vi "cameraParameters.vi"(2 "Camera Device  IN":T2, 3 "Camera Parameters":refnum<vi>, 4 "Selector":refnum<vi>, 5 "Stream?":refnum<vi>) -> (0 "Camera Device OUT":T1, 1 "Stream? OUT":bool)   [LabVIEW 2010]
uses:
  <vilib>/addons/PixeLINK/Low Level Functions/CAMERA_FEATURES.llb/TDPU-CameraFeatures-PixelFormat.ctl
  <vilib>/Utility/error.llb/DialogType.ctl
  <vilib>/addons/PixeLINK/Low Level Functions/CAMERA_FEATURES.llb/TDPU-CameraFeatures-FeatureFlags.ctl
  <vilib>/addons/PixeLINK/Low Level Functions/CAMERA_FEATURES.llb/TDPU-CameraFeatures-FeatureIds.ctl
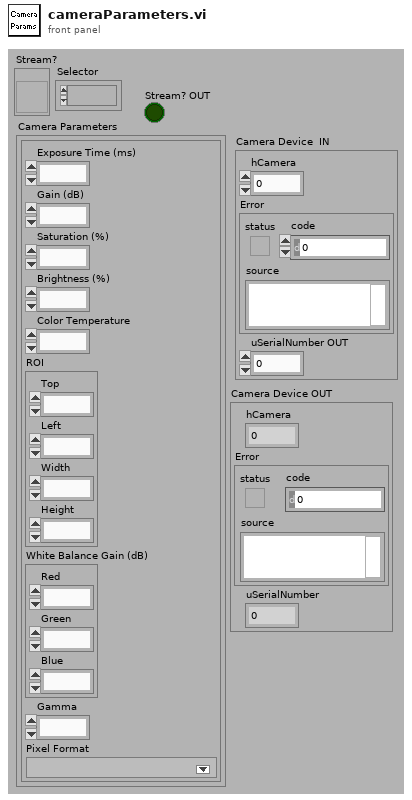
[diagram p1: front panel]
types:
  T1 = cluster{"hCamera":u32, "Error":errorcluster, "uSerialNumber":u32}
  T2 = cluster{"hCamera":u32, "Error":errorcluster, "uSerialNumber OUT":u32}
  T3 = typedef "TDPU-CameraFeatures-PixelFormat.ctl" = u16
  T4 = cluster{"Selector":u16, "Stream?":bool, "Camera Parameters":cluster{"Exposure Time (ms)":u32, "Gain (dB)":dbl, "Saturation (%)":dbl, "Brightness (%)":dbl, "Color Temperature":dbl, "ROI":cluster{"Top":i32, "Left":i32, "Width":i32, "Height":i32}, "White Balance Gain (dB)":cluster{"Red":dbl, "Green":dbl, "Blue":dbl}, "Gamma":dbl, "Pixel Format":T3}}
  T5 = cluster{"Exposure Time (ms)":u32, "Gain (dB)":dbl, "Saturation (%)":dbl, "Brightness (%)":dbl, "Color Temperature":dbl, "ROI":cluster{"Top":i32, "Left":i32, "Width":i32, "Height":i32}, "White Balance Gain (dB)":cluster{"Red":dbl, "Green":dbl, "Blue":dbl}, "Gamma":dbl, "Pixel Format":T3}
  T6 = cluster{"Exposure Time (ms)":dbl, "Gain (dB)":dbl, "Saturation (%)":dbl, "Brightness (%)":dbl, "Color Temperature":dbl, "ROI":cluster{"Top":i32, "Left":i32, "Width":i32, "Height":i32}, "White Balance Gain (dB)":cluster{"Red":dbl, "Green":dbl, "Blue":dbl}, "Gamma":dbl, "Pixel Format":T3}
  T7 = typedef "DialogType.ctl" = u16
  T8 = enum16{"Exposure Time (ms)", "Gain (dB)", "Saturation (%)", "Brightness (%)", "Color Temperature (%)", "ROI", "White Balance Gain (dB)", "Gamma", "Pixel Format", "Selector", "Stream", "Nothing"}[]
  T9 = typedef "TDPU-CameraFeatures-FeatureFlags.ctl" = u32
  T10 = typedef "TDPU-CameraFeatures-FeatureIds.ctl" = u32
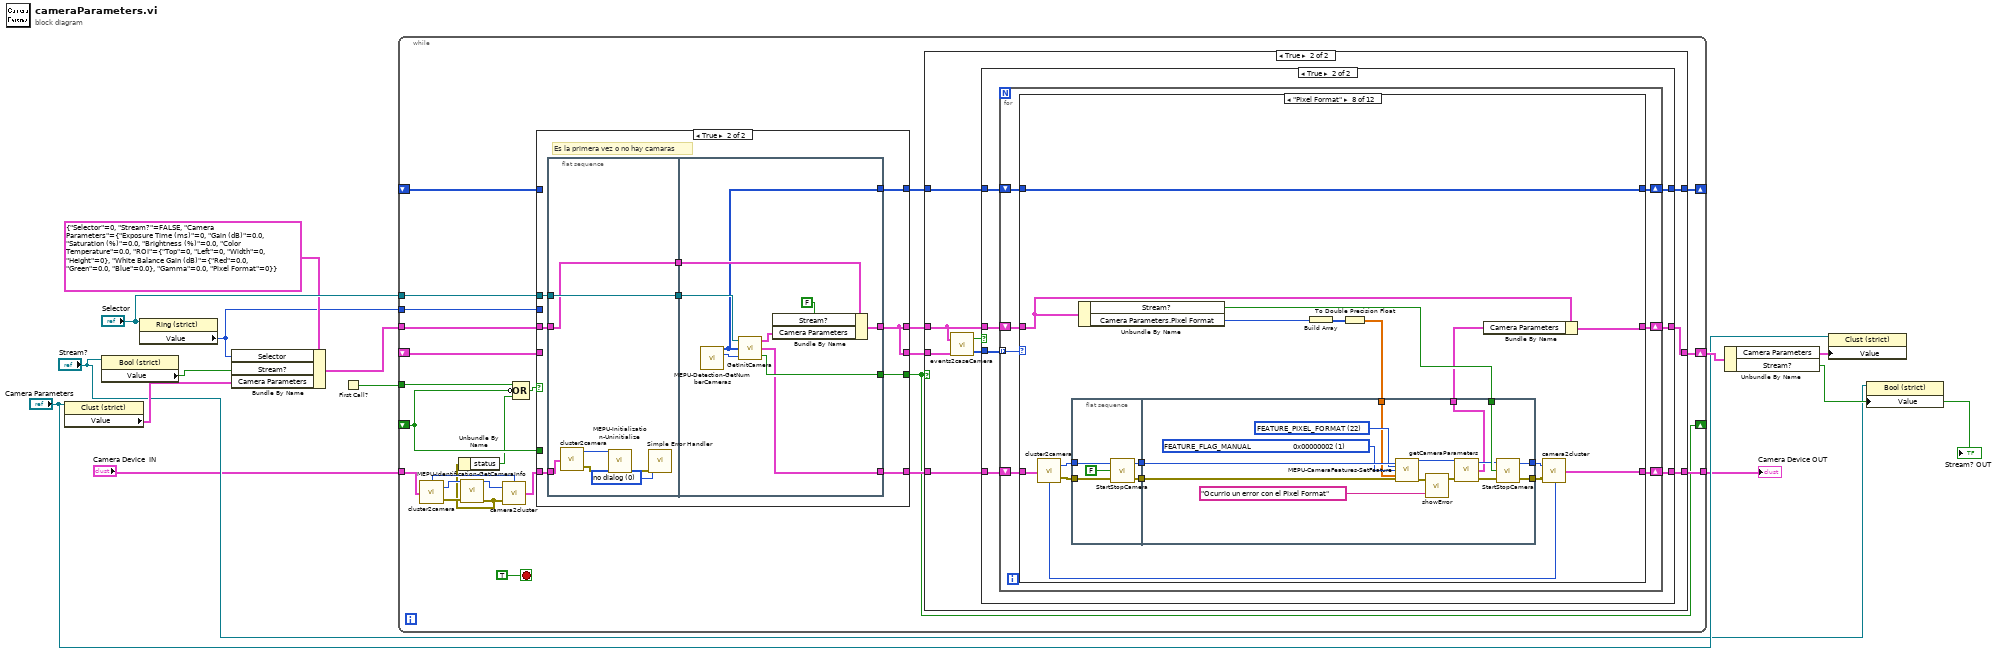
[diagram p0: block diagram]
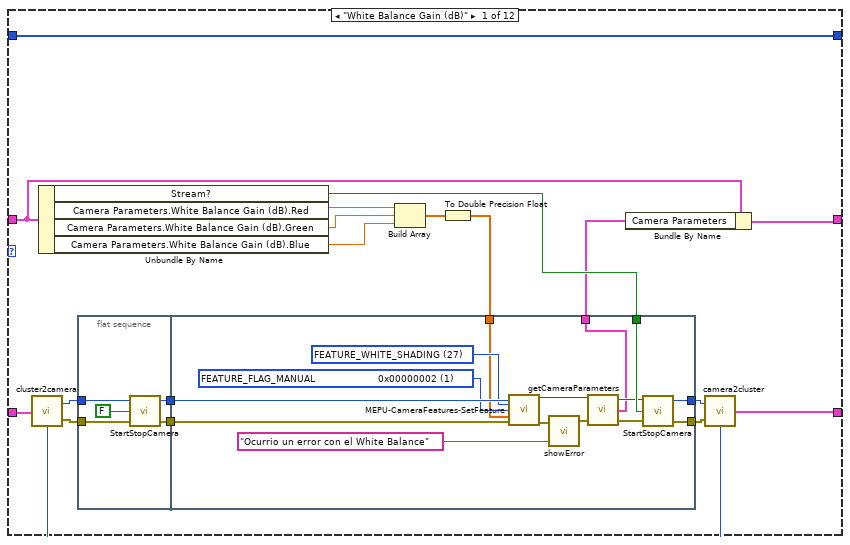
[diagram p4: hidden frame]
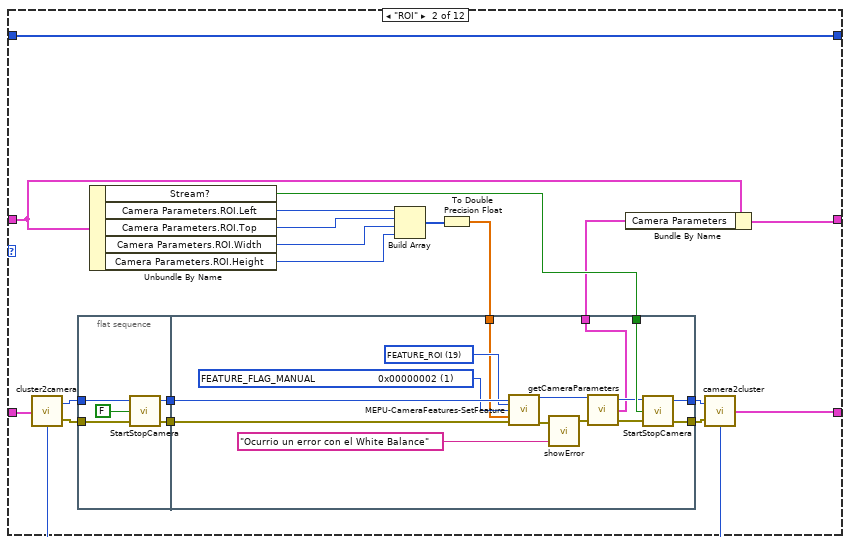
[diagram p5: hidden frame]
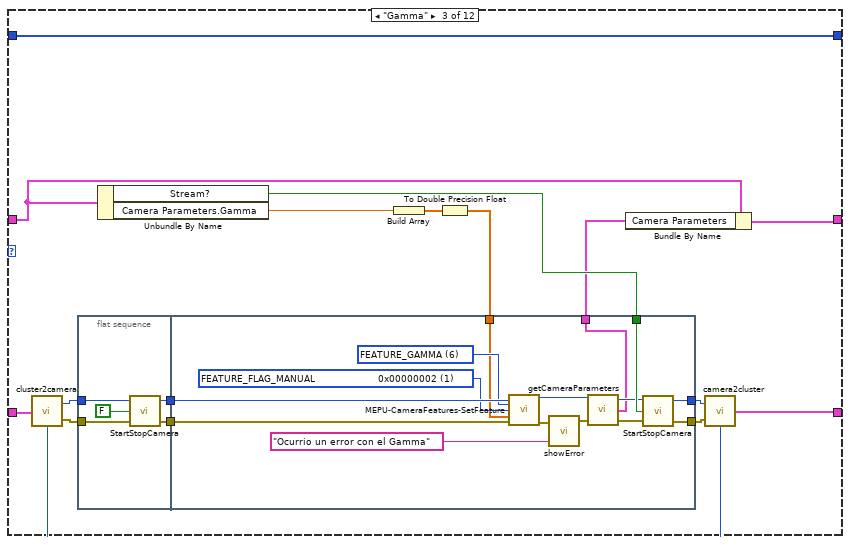
[diagram p6: hidden frame]
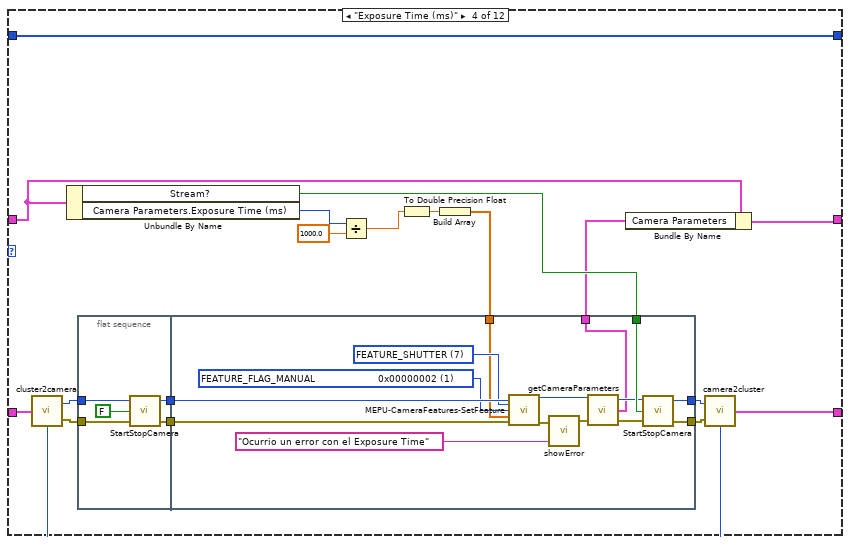
[diagram p7: hidden frame]
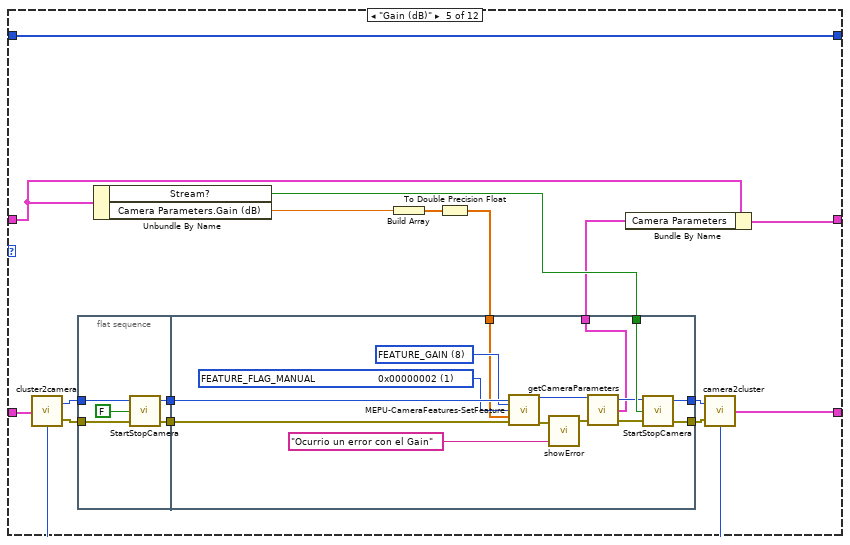
[diagram p8: hidden frame]
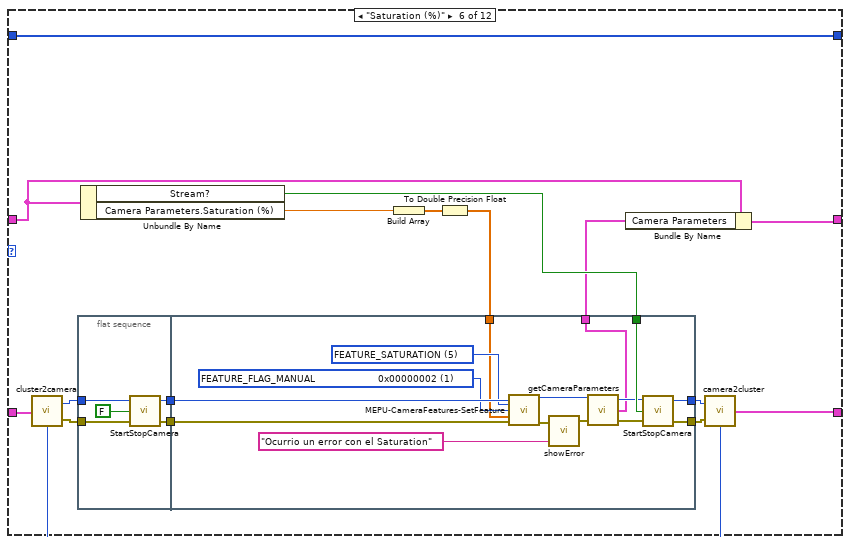
[diagram p9: hidden frame]
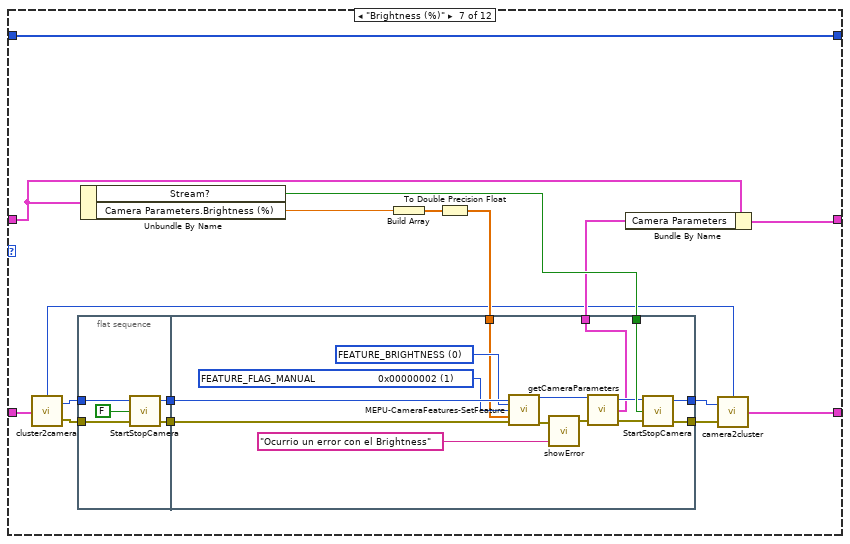
[diagram p10: hidden frame]
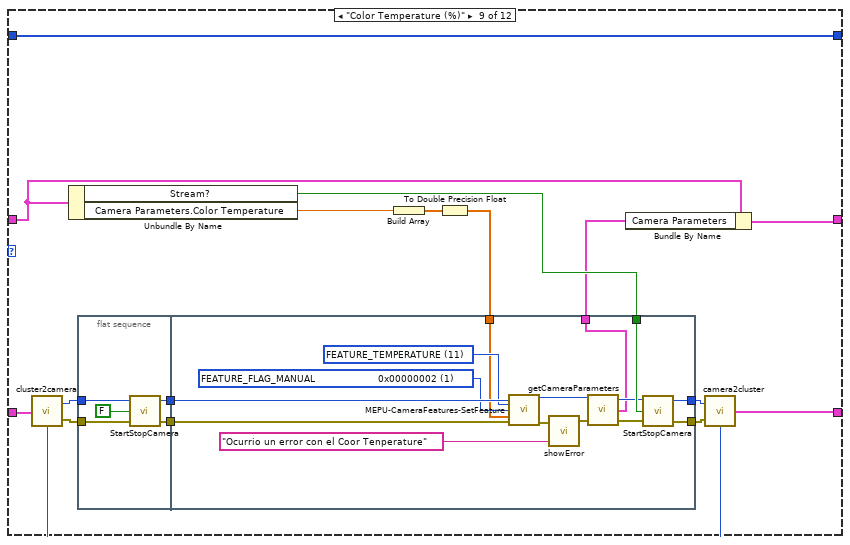
[diagram p11: hidden frame]
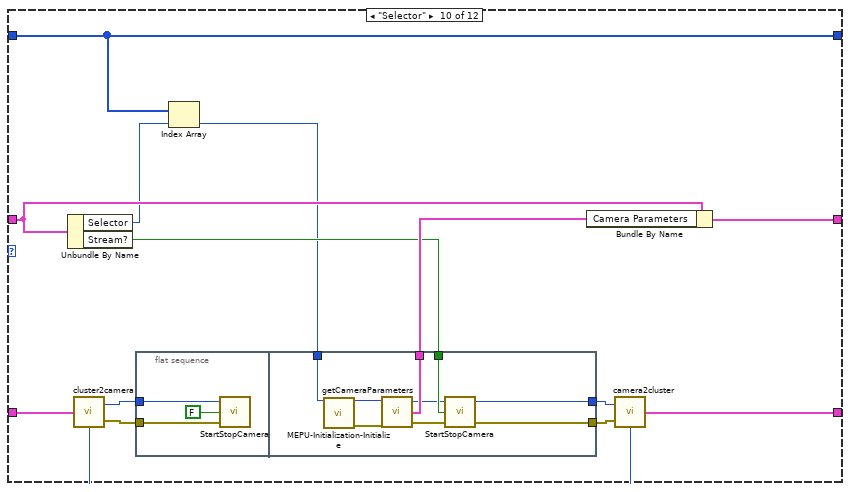
[diagram p12: hidden frame]
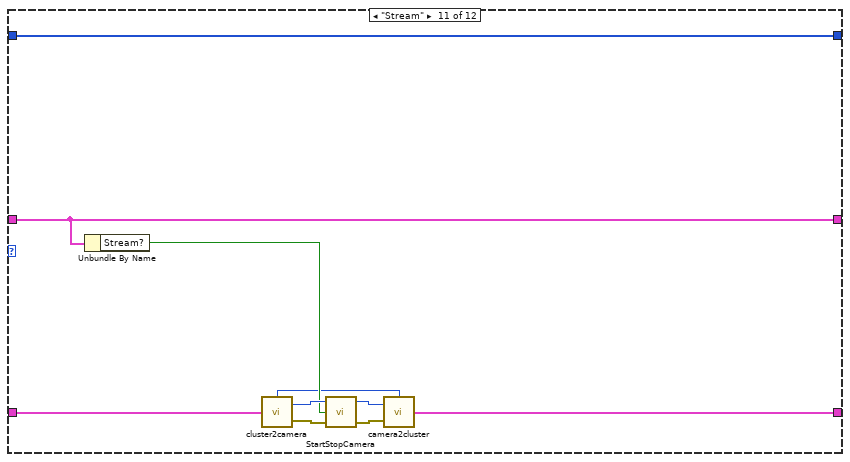
[diagram p13: hidden frame]
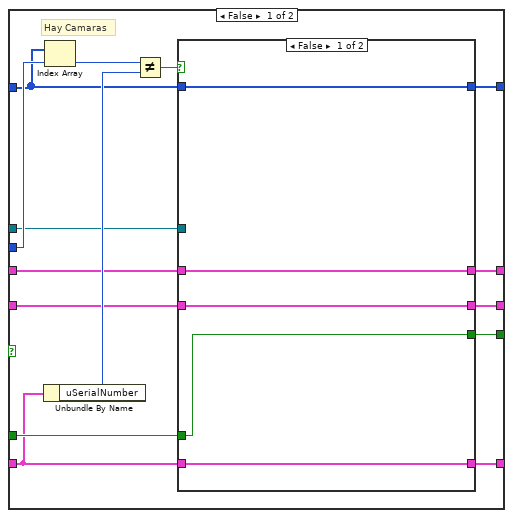
[diagram p15: hidden frame]
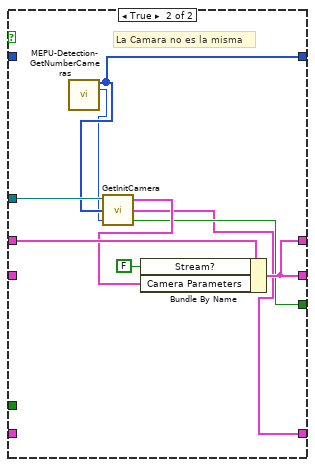
[diagram p16: hidden frame]
diagram:
  n1 = property class="Clust (strict)"(reference="Camera Parameters") -> ("Value"=w7:T5)  [unwired: 1 in, 2 out]
  n2 = property class="Bool (strict)"(reference="Stream?") -> ("Value"=w6:bool)  [unwired: 1 in, 2 out]
  n3 = property class="Ring (strict)"(reference="Selector") -> ("Value"=w3:u16)  [unwired: 1 in, 2 out]
  n4 = Bundle By Name(cluster=T4 {"Selector"=0, "Stream?"=FALSE, "Camera Parameters"={"Exposure Time (ms)"=0, "Gain (dB)"=0.0, "Saturation (%)"=0.0, "Brightness (%)"=0.0, "Color Temperature"=0.0, "ROI"={"Top"=0, "Left"=0, "Width"=0, "Height"=0}, "White Balance Gain (dB)"={"Red"=0.0, "Green"=0.0, "Blue"=0.0}, "Gamma"=0.0, "Pixel Format"=0}}, "Selector"=w3, "Stream?"=w6, "Camera Parameters"=w7) -> (w13:T4)
  n5 = First Call?() -> (First Call?: T/F=w14:bool)
  n6 = while {
    tunnel: w13 -> [w35]
    shift-right: [w38] -> w12
    shift-left: _ -> [w34]
    tunnel: "Camera Device  IN" -> [w18]
    tunnel: [w37] -> w1
    tunnel: w14 -> [w25]
    tunnel: "Selector" -> [w31]
    shift-right: [w27] -> _
    shift-left: _ -> [w30]
    shift-right: [w26] -> _
    shift-left: _ -> [w23]
    tunnel: w3 -> [w24]
    stop <- TRUE stop-if-true
    n7 = call "cluster2camera.vi"("Camera Device IN"=w18) -> ("Error OUT"=w22:errorcluster, "hCamera OUT"=w21:u32, "uSerialNumber OUT"=w19:u32)  [unwired: 2 in]
    n8 = call <vilib>:"MEPU-Identification-GetCameraInfo.vi"("hCamera IN"=w21, "Error IN"=w22) -> ("hCamera OUT"=w20:u32, "Error OUT"=w16:errorcluster)  [unwired: 11 in, 1 out]
    n9 = Unbundle By Name(w16) -> ("status"=w15:bool)
    n10 = call "camera2cluster.vi"("uSerialNumber IN"=w19, "Error IN"=w16, "hCamera IN"=w20) -> ("Camera Device OUT"=w17:T1)
    n11 = Compound Arithmetic op=OR(w25, invert w23, w15) -> (w29:bool)
    n12 = case shown="True" w29 {
      tunnel: [w458 w477] -> w28
      tunnel: [w456 w478] -> w36
      tunnel: w35 -> [w455 w480]
      tunnel: w34 -> [w453 _]
      tunnel: [w454 w478] -> w33
      tunnel: [w450 w481] -> w32
      tunnel: w17 -> [w449 w485]
      tunnel: w30 -> [w457 _]
      tunnel: [w452 w482] -> w26
      tunnel: w31 -> [w448 w483]
      tunnel: w24 -> [w462 _]
      tunnel: w23 -> [w451 _]
      frame False {
        # "Hay Camaras"
        n13 = Unbundle By Name(w449) -> ("uSerialNumber"=w460:u32)
        n14 = Index Array(array=w457, index=w462) -> (element=w461:u32)
        n15 = Not Equal?(x=w461, y=w460) -> (x != y?=w459:bool)
        n16 = case shown="False" w459 {
          tunnel: [w463 w475] -> w458
          tunnel: w457 -> [w463 _]
          tunnel: [w464 w472] -> w456
          tunnel: w455 -> [w464 w473]
          tunnel: [w465 w472] -> w454
          tunnel: w453 -> [w465 _]
          tunnel: [w466 w469] -> w452
          tunnel: w451 -> [w466 _]
          tunnel: [w467 w468] -> w450
          tunnel: w449 -> [w467 _]
          tunnel: w448 -> [_ w476]
          frame False {
          }
          frame True {
            # "La Camara no es la misma"
            n17 = call <vilib>:"MEPU-Detection-GetNumberCameras.vi"() -> ("LV_SerialNumbers OUT"=w475:u32[], "LV_NumberSerial OUT"=w474:u32)  [unwired: 13 in, 1 out]
            n18 = call "GetInitCamera.vi"("LV_NumberSerial IN"=w474, "LV_SerialNumbers IN"=w475, "Selector"=w476) -> ("Hay Camaras?"=w469:bool, "Camera Device OUT"=w468:T2, "Camera Parameters OUT"=w470:T6)
            n19 = Bundle By Name(cluster=w473, "Stream?"=FALSE, "Camera Parameters"=w470) -> (w472:T4)
          }
        }
      }
      frame True {
        # "Es la primera vez o no hay camaras"
        n20 = flat-sequence {
          tunnel: w485 -> [w488]
          tunnel: [w487] -> w484
          tunnel: w483 -> [w487]
          tunnel: w480 -> [w486]
          tunnel: [w486] -> w479
          tunnel: w484 -> [w500]
          tunnel: [w498] -> w482
          tunnel: [w497] -> w481
          tunnel: w479 -> [w495]
          tunnel: [w494] -> w478
          tunnel: [w493] -> w477
          frame #0 {
            w489 = T7 0 items=["no dialog", "OK message", "continue or stop message", "OK message + warnings", "continue/stop + warnings"] ("type of dialog (OK msg:1)")
            n21 = call "cluster2camera.vi"("Camera Device IN"=w488) -> ("Error OUT"=w492:errorcluster, "hCamera OUT"=w491:u32)  [unwired: 2 in, 1 out]
            n22 = call <vilib>:"MEPU-Initialization-Uninitialize.vi"("hCamera IN"=w491, "Error IN"=w492) -> ("Error OUT"=w490:errorcluster)  [unwired: 13 in]
            n23 = call <vilib>:"Simple Error Handler.vi"("type of dialog (OK msg:1)"=w489, "error in (no error)"=w490) -> ()  [unwired: 3 in, 5 out]
          }
          frame #1 {
            n24 = call <vilib>:"MEPU-Detection-GetNumberCameras.vi"() -> ("LV_SerialNumbers OUT"=w493:u32[], "LV_NumberSerial OUT"=w499:u32)  [unwired: 13 in, 1 out]
            n25 = call "GetInitCamera.vi"("LV_NumberSerial IN"=w499, "LV_SerialNumbers IN"=w493, "Selector"=w500) -> ("Hay Camaras?"=w498:bool, "Camera Device OUT"=w497:T2, "Camera Parameters OUT"=w496:T6)
            n26 = Bundle By Name(cluster=w495, "Stream?"=FALSE, "Camera Parameters"=w496) -> (w494:T4)
          }
        }
      }
    }
    n27 = case shown="True" w26 {
      tunnel: [w42 w50] -> w38
      tunnel: [w41 w48] -> w37
      tunnel: w28 -> [w40 w47]
      tunnel: w36 -> [w42 w46]
      tunnel: w33 -> [_ w45]
      tunnel: w32 -> [w41 w44]
      tunnel: [w40 w43] -> w27
      frame False {
      }
      frame True {
        n28 = call "events2caseCamera.vi"("Camara Controls Old"=w45, "Camara Controls New"=w46) -> ("Cameara Cambio Array"=w49:T8, "Camara Cambio?"=w51:bool)
        n29 = case shown="True" w51 {
          tunnel: [w54 w59] -> w50
          tunnel: w46 -> [w54 w60]
          tunnel: w49 -> [_ w61]
          tunnel: w44 -> [w53 w58]
          tunnel: [w53 w57] -> w48
          tunnel: w47 -> [w52 w56]
          tunnel: [w52 w55] -> w43
          frame False {
          }
          frame True {
            n30 = for {
              tunnel: w61 -> [w68] mode=indexing
              shift-right: [w66] -> w59
              shift-left: w60 -> [w67]
              shift-right: [w64] -> w57
              shift-left: w58 -> [w65]
              shift-right: [w63] -> w55
              shift-left: w56 -> [w62]
              n31 = case shown="\"Pixel Format\"" w68 {
                tunnel: w67 -> [w79 w119 w156 w195 w232 w269 w308 w343 w380 w421 w443 w447]
                tunnel: [w80 w120 w157 w196 w233 w270 w309 w344 w381 w422 w443 w447] -> w66
                tunnel: w65 -> [w71 w108 w150 w186 w225 w262 w299 w336 w374 w411 w437 w446]
                tunnel: [w70 w109 w149 w187 w226 w263 w300 w337 w372 w410 w436 w446] -> w64
                tunnel: [w74 w114 w153 w193 w229 w266 w305 w340 w377 w415 w444 w445] -> w63
                tunnel: w62 -> [w74 w114 w153 w193 w229 w266 w305 w340 w377 w415 w444 w445]
                frame "White Balance Gain (dB)" {
                  n32 = call "cluster2camera.vi"("Camera Device IN"=w71) -> ("Error OUT"=w84:errorcluster, "hCamera OUT"=w85:u32, "uSerialNumber OUT"=w69:u32)  [unwired: 2 in]
                  n33 = Unbundle By Name(w79) -> ("Stream?"=w81:bool, "Camera Parameters.White Balance Gain (dB).Red"=w78:dbl, "Camera Parameters.White Balance Gain (dB).Green"=w77:dbl, "Camera Parameters.White Balance Gain (dB).Blue"=w76:dbl)
                  n34 = flat-sequence {
                    tunnel: w85 -> [w91]
                    tunnel: w84 -> [w90]
                    tunnel: [w89] -> w87
                    tunnel: [w88] -> w86
                    tunnel: w81 -> [w107]
                    tunnel: [w106] -> w83
                    tunnel: [w105] -> w82
                    tunnel: w87 -> [w104]
                    tunnel: w86 -> [w103]
                    tunnel: [w97] -> w75
                    tunnel: w72 -> [w96]
                    frame #0 {
                      n35 = call "StartStopCamera.vi"("Error IN"=w90, "Camara ON?"=FALSE, "hCamera IN"=w91) -> ("Error OUT"=w88:errorcluster, "hCamera OUT"=w89:u32)  [unwired: 1 in]
                    }
                    frame #1 {
                      w101 = T9 1 items=["FEATURE_FLAG_PRESENCE                 0x00000001", "FEATURE_FLAG_MANUAL                     0x00000002", "FEATURE_FLAG_AUTO                         0x00000004", "FEATURE_FLAG_ONEPUSH                   0x00000008", "FEATURE_FLAG_OFF                            0x00000010", "FEATURE_FLAG_DESC_SUPPORTED    0x00000020", "FEATURE_FLAG_READ_ONLY               0x00000040"] ("uFlags IN")
                      w102 = T10 27 items=["FEATURE_BRIGHTNESS", "FEATURE_EXPOSURE", "FEATURE_SHARPNESS", "FEATURE_WHITE_BAL", "FEATURE_HUE", "FEATURE_SATURATION", "FEATURE_GAMMA", "FEATURE_SHUTTER", "FEATURE_GAIN", "FEATURE_IRIS", "FEATURE_FOCUS", "FEATURE_TEMPERATURE", "FEATURE_TRIGGER", "FEATURE_ZOOM", "FEATURE_PAN", "FEATURE_TILT", "FEATURE_OPT_FILTER", "FEATURE_GPIO", "FEATURE_FRAME_RATE", "FEATURE_ROI", "FEATURE_FLIP", "FEATURE_PIXEL_ADDRESSING", "FEATURE_PIXEL_FORMAT", "FEATURE_EXTENDED_SHUTTER", "FEATURE_AUTO_ROI", "FEATURE_LOOKUP_TABLE", "FEATURE_MEMORY_CHANNEL", "FEATURE_WHITE_SHADING", "FEATURE_ROTATE", "FEATURE_IMAGER_CLK_DIVISOR", "FEATURE_TRIG_WITH_CNTRLD_LIGHT", "FEATURE_MAX_PIXEL_SIZE"] ("uFeatureId IN")
                      n36 = call <vilib>:"MEPU-CameraFeatures-SetFeature.vi"("hCamera IN"=w104, "uFeatureId IN"=w102, "uFlags IN"=w101, "pParms IN"=w96, "Error IN"=w103) -> ("hCamera OUT"=w100:u32, "Error OUT"=w95:errorcluster)  [unwired: 8 in, 1 out]
                      n37 = call "showError.vi"("message"="Ocurrio un error con el White Balance", "Error IN"=w95) -> ("Error OUT"=w94:errorcluster)  [unwired: 3 in]
                      n38 = call "getCameraParameters.vi"("Error IN"=w94, "hCamera IN"=w100) -> ("Error OUT"=w98:errorcluster, "Camera Parameters"=w97:T6, "hCamera OUT"=w99:u32)  [unwired: 1 in]
                      n39 = call "StartStopCamera.vi"("Error IN"=w98, "Camara ON?"=w107, "hCamera IN"=w99) -> ("Error OUT"=w105:errorcluster, "hCamera OUT"=w106:u32)  [unwired: 1 in]
                    }
                  }
                  n40 = Build Array(w78, w77, w76) -> (w73:dbl[])
                  n41 = To Double Precision Float(number=w73) -> (double precision float=w72:dbl[])
                  n42 = Bundle By Name(cluster=w79, "Camera Parameters"=w75) -> (w80:T4)
                  n43 = call "camera2cluster.vi"("uSerialNumber IN"=w69, "Error IN"=w82, "hCamera IN"=w83) -> ("Camera Device OUT"=w70:T1)
                }
                frame "ROI" {
                  n44 = call "cluster2camera.vi"("Camera Device IN"=w108) -> ("Error OUT"=w124:errorcluster, "hCamera OUT"=w125:u32, "uSerialNumber OUT"=w110:u32)  [unwired: 2 in]
                  n45 = flat-sequence {
                    tunnel: w125 -> [w131]
                    tunnel: w124 -> [w130]
                    tunnel: [w129] -> w127
                    tunnel: [w128] -> w126
                    tunnel: w121 -> [w147]
                    tunnel: [w146] -> w123
                    tunnel: [w145] -> w122
                    tunnel: w127 -> [w144]
                    tunnel: w126 -> [w143]
                    tunnel: [w137] -> w115
                    tunnel: w111 -> [w136]
                    frame #0 {
                      n46 = call "StartStopCamera.vi"("Error IN"=w130, "Camara ON?"=FALSE, "hCamera IN"=w131) -> ("Error OUT"=w128:errorcluster, "hCamera OUT"=w129:u32)  [unwired: 1 in]
                    }
                    frame #1 {
                      w141 = T9 1 items=["FEATURE_FLAG_PRESENCE                 0x00000001", "FEATURE_FLAG_MANUAL                     0x00000002", "FEATURE_FLAG_AUTO                         0x00000004", "FEATURE_FLAG_ONEPUSH                   0x00000008", "FEATURE_FLAG_OFF                            0x00000010", "FEATURE_FLAG_DESC_SUPPORTED    0x00000020", "FEATURE_FLAG_READ_ONLY               0x00000040"] ("uFlags IN")
                      w142 = T10 19 items=["FEATURE_BRIGHTNESS", "FEATURE_EXPOSURE", "FEATURE_SHARPNESS", "FEATURE_WHITE_BAL", "FEATURE_HUE", "FEATURE_SATURATION", "FEATURE_GAMMA", "FEATURE_SHUTTER", "FEATURE_GAIN", "FEATURE_IRIS", "FEATURE_FOCUS", "FEATURE_TEMPERATURE", "FEATURE_TRIGGER", "FEATURE_ZOOM", "FEATURE_PAN", "FEATURE_TILT", "FEATURE_OPT_FILTER", "FEATURE_GPIO", "FEATURE_FRAME_RATE", "FEATURE_ROI", "FEATURE_FLIP", "FEATURE_PIXEL_ADDRESSING", "FEATURE_PIXEL_FORMAT", "FEATURE_EXTENDED_SHUTTER", "FEATURE_AUTO_ROI", "FEATURE_LOOKUP_TABLE", "FEATURE_MEMORY_CHANNEL", "FEATURE_WHITE_SHADING", "FEATURE_ROTATE", "FEATURE_IMAGER_CLK_DIVISOR", "FEATURE_TRIG_WITH_CNTRLD_LIGHT", "FEATURE_MAX_PIXEL_SIZE"] ("uFeatureId IN")
                      n47 = call <vilib>:"MEPU-CameraFeatures-SetFeature.vi"("hCamera IN"=w144, "uFeatureId IN"=w142, "uFlags IN"=w141, "pParms IN"=w136, "Error IN"=w143) -> ("hCamera OUT"=w140:u32, "Error OUT"=w135:errorcluster)  [unwired: 8 in, 1 out]
                      n48 = call "showError.vi"("message"="Ocurrio un error con el White Balance", "Error IN"=w135) -> ("Error OUT"=w134:errorcluster)  [unwired: 3 in]
                      n49 = call "getCameraParameters.vi"("Error IN"=w134, "hCamera IN"=w140) -> ("Error OUT"=w138:errorcluster, "Camera Parameters"=w137:T6, "hCamera OUT"=w139:u32)  [unwired: 1 in]
                      n50 = call "StartStopCamera.vi"("Error IN"=w138, "Camara ON?"=w147, "hCamera IN"=w139) -> ("Error OUT"=w145:errorcluster, "hCamera OUT"=w146:u32)  [unwired: 1 in]
                    }
                  }
                  n51 = Unbundle By Name(w119) -> ("Stream?"=w121:bool, "Camera Parameters.ROI.Left"=w118:i32, "Camera Parameters.ROI.Top"=w117:i32, "Camera Parameters.ROI.Width"=w116:i32, "Camera Parameters.ROI.Height"=w113:i32)
                  n52 = Build Array(w118, w117, w116, w113) -> (w112:i32[])
                  n53 = To Double Precision Float(number=w112) -> (double precision float=w111:dbl[])
                  n54 = Bundle By Name(cluster=w119, "Camera Parameters"=w115) -> (w120:T4)
                  n55 = call "camera2cluster.vi"("uSerialNumber IN"=w110, "Error IN"=w122, "hCamera IN"=w123) -> ("Camera Device OUT"=w109:T1)
                }
                frame "Gamma" {
                  n56 = call "cluster2camera.vi"("Camera Device IN"=w150) -> ("Error OUT"=w161:errorcluster, "hCamera OUT"=w162:u32, "uSerialNumber OUT"=w148:u32)  [unwired: 2 in]
                  n57 = flat-sequence {
                    tunnel: w162 -> [w168]
                    tunnel: w161 -> [w167]
                    tunnel: [w166] -> w164
                    tunnel: [w165] -> w163
                    tunnel: w158 -> [w184]
                    tunnel: [w183] -> w160
                    tunnel: [w182] -> w159
                    tunnel: w164 -> [w181]
                    tunnel: w163 -> [w180]
                    tunnel: [w174] -> w154
                    tunnel: w151 -> [w173]
                    frame #0 {
                      n58 = call "StartStopCamera.vi"("Error IN"=w167, "Camara ON?"=FALSE, "hCamera IN"=w168) -> ("Error OUT"=w165:errorcluster, "hCamera OUT"=w166:u32)  [unwired: 1 in]
                    }
                    frame #1 {
                      w178 = T9 1 items=["FEATURE_FLAG_PRESENCE                 0x00000001", "FEATURE_FLAG_MANUAL                     0x00000002", "FEATURE_FLAG_AUTO                         0x00000004", "FEATURE_FLAG_ONEPUSH                   0x00000008", "FEATURE_FLAG_OFF                            0x00000010", "FEATURE_FLAG_DESC_SUPPORTED    0x00000020", "FEATURE_FLAG_READ_ONLY               0x00000040"] ("uFlags IN")
                      w179 = T10 6 items=["FEATURE_BRIGHTNESS", "FEATURE_EXPOSURE", "FEATURE_SHARPNESS", "FEATURE_WHITE_BAL", "FEATURE_HUE", "FEATURE_SATURATION", "FEATURE_GAMMA", "FEATURE_SHUTTER", "FEATURE_GAIN", "FEATURE_IRIS", "FEATURE_FOCUS", "FEATURE_TEMPERATURE", "FEATURE_TRIGGER", "FEATURE_ZOOM", "FEATURE_PAN", "FEATURE_TILT", "FEATURE_OPT_FILTER", "FEATURE_GPIO", "FEATURE_FRAME_RATE", "FEATURE_ROI", "FEATURE_FLIP", "FEATURE_PIXEL_ADDRESSING", "FEATURE_PIXEL_FORMAT", "FEATURE_EXTENDED_SHUTTER", "FEATURE_AUTO_ROI", "FEATURE_LOOKUP_TABLE", "FEATURE_MEMORY_CHANNEL", "FEATURE_WHITE_SHADING", "FEATURE_ROTATE", "FEATURE_IMAGER_CLK_DIVISOR", "FEATURE_TRIG_WITH_CNTRLD_LIGHT", "FEATURE_MAX_PIXEL_SIZE"] ("uFeatureId IN")
                      n59 = call <vilib>:"MEPU-CameraFeatures-SetFeature.vi"("hCamera IN"=w181, "uFeatureId IN"=w179, "uFlags IN"=w178, "pParms IN"=w173, "Error IN"=w180) -> ("hCamera OUT"=w177:u32, "Error OUT"=w172:errorcluster)  [unwired: 8 in, 1 out]
                      n60 = call "showError.vi"("message"="Ocurrio un error con el Gamma", "Error IN"=w172) -> ("Error OUT"=w171:errorcluster)  [unwired: 3 in]
                      n61 = call "getCameraParameters.vi"("Error IN"=w171, "hCamera IN"=w177) -> ("Error OUT"=w175:errorcluster, "Camera Parameters"=w174:T6, "hCamera OUT"=w176:u32)  [unwired: 1 in]
                      n62 = call "StartStopCamera.vi"("Error IN"=w175, "Camara ON?"=w184, "hCamera IN"=w176) -> ("Error OUT"=w182:errorcluster, "hCamera OUT"=w183:u32)  [unwired: 1 in]
                    }
                  }
                  n63 = Unbundle By Name(w156) -> ("Stream?"=w158:bool, "Camera Parameters.Gamma"=w155:dbl)
                  n64 = Build Array(w155) -> (w152:dbl[])
                  n65 = To Double Precision Float(number=w152) -> (double precision float=w151:dbl[])
                  n66 = Bundle By Name(cluster=w156, "Camera Parameters"=w154) -> (w157:T4)
                  n67 = call "camera2cluster.vi"("uSerialNumber IN"=w148, "Error IN"=w159, "hCamera IN"=w160) -> ("Camera Device OUT"=w149:T1)
                }
                frame "Exposure Time (ms)" {
                  n68 = call "cluster2camera.vi"("Camera Device IN"=w186) -> ("Error OUT"=w200:errorcluster, "hCamera OUT"=w201:u32, "uSerialNumber OUT"=w185:u32)  [unwired: 2 in]
                  n69 = Unbundle By Name(w195) -> ("Stream?"=w197:bool, "Camera Parameters.Exposure Time (ms)"=w192:u32)
                  n70 = flat-sequence {
                    tunnel: w201 -> [w207]
                    tunnel: w200 -> [w206]
                    tunnel: [w205] -> w203
                    tunnel: [w204] -> w202
                    tunnel: w197 -> [w223]
                    tunnel: [w222] -> w199
                    tunnel: [w221] -> w198
                    tunnel: w203 -> [w220]
                    tunnel: w202 -> [w219]
                    tunnel: [w213] -> w194
                    tunnel: w190 -> [w212]
                    frame #0 {
                      n71 = call "StartStopCamera.vi"("Error IN"=w206, "Camara ON?"=FALSE, "hCamera IN"=w207) -> ("Error OUT"=w204:errorcluster, "hCamera OUT"=w205:u32)  [unwired: 1 in]
                    }
                    frame #1 {
                      w217 = T9 1 items=["FEATURE_FLAG_PRESENCE                 0x00000001", "FEATURE_FLAG_MANUAL                     0x00000002", "FEATURE_FLAG_AUTO                         0x00000004", "FEATURE_FLAG_ONEPUSH                   0x00000008", "FEATURE_FLAG_OFF                            0x00000010", "FEATURE_FLAG_DESC_SUPPORTED    0x00000020", "FEATURE_FLAG_READ_ONLY               0x00000040"] ("uFlags IN")
                      w218 = T10 7 items=["FEATURE_BRIGHTNESS", "FEATURE_EXPOSURE", "FEATURE_SHARPNESS", "FEATURE_WHITE_BAL", "FEATURE_HUE", "FEATURE_SATURATION", "FEATURE_GAMMA", "FEATURE_SHUTTER", "FEATURE_GAIN", "FEATURE_IRIS", "FEATURE_FOCUS", "FEATURE_TEMPERATURE", "FEATURE_TRIGGER", "FEATURE_ZOOM", "FEATURE_PAN", "FEATURE_TILT", "FEATURE_OPT_FILTER", "FEATURE_GPIO", "FEATURE_FRAME_RATE", "FEATURE_ROI", "FEATURE_FLIP", "FEATURE_PIXEL_ADDRESSING", "FEATURE_PIXEL_FORMAT", "FEATURE_EXTENDED_SHUTTER", "FEATURE_AUTO_ROI", "FEATURE_LOOKUP_TABLE", "FEATURE_MEMORY_CHANNEL", "FEATURE_WHITE_SHADING", "FEATURE_ROTATE", "FEATURE_IMAGER_CLK_DIVISOR", "FEATURE_TRIG_WITH_CNTRLD_LIGHT", "FEATURE_MAX_PIXEL_SIZE"] ("uFeatureId IN")
                      n72 = call <vilib>:"MEPU-CameraFeatures-SetFeature.vi"("hCamera IN"=w220, "uFeatureId IN"=w218, "uFlags IN"=w217, "pParms IN"=w212, "Error IN"=w219) -> ("hCamera OUT"=w216:u32, "Error OUT"=w211:errorcluster)  [unwired: 8 in, 1 out]
                      n73 = call "showError.vi"("message"="Ocurrio un error con el Exposure Time", "Error IN"=w211) -> ("Error OUT"=w210:errorcluster)  [unwired: 3 in]
                      n74 = call "getCameraParameters.vi"("Error IN"=w210, "hCamera IN"=w216) -> ("Error OUT"=w214:errorcluster, "Camera Parameters"=w213:T6, "hCamera OUT"=w215:u32)  [unwired: 1 in]
                      n75 = call "StartStopCamera.vi"("Error IN"=w214, "Camara ON?"=w223, "hCamera IN"=w215) -> ("Error OUT"=w221:errorcluster, "hCamera OUT"=w222:u32)  [unwired: 1 in]
                    }
                  }
                  n76 = Divide(x=w192, y=1000.0) -> (x/y=w189:dbl)
                  n77 = To Double Precision Float(number=w189) -> (double precision float=w188:dbl)
                  n78 = Build Array(w188) -> (w190:dbl[])
                  n79 = Bundle By Name(cluster=w195, "Camera Parameters"=w194) -> (w196:T4)
                  n80 = call "camera2cluster.vi"("uSerialNumber IN"=w185, "Error IN"=w198, "hCamera IN"=w199) -> ("Camera Device OUT"=w187:T1)
                }
                frame "Gain (dB)" {
                  n81 = call "cluster2camera.vi"("Camera Device IN"=w225) -> ("Error OUT"=w237:errorcluster, "hCamera OUT"=w238:u32, "uSerialNumber OUT"=w224:u32)  [unwired: 2 in]
                  n82 = flat-sequence {
                    tunnel: w238 -> [w244]
                    tunnel: w237 -> [w243]
                    tunnel: [w242] -> w240
                    tunnel: [w241] -> w239
                    tunnel: w234 -> [w260]
                    tunnel: [w259] -> w236
                    tunnel: [w258] -> w235
                    tunnel: w240 -> [w257]
                    tunnel: w239 -> [w256]
                    tunnel: [w250] -> w230
                    tunnel: w227 -> [w249]
                    frame #0 {
                      n83 = call "StartStopCamera.vi"("Error IN"=w243, "Camara ON?"=FALSE, "hCamera IN"=w244) -> ("Error OUT"=w241:errorcluster, "hCamera OUT"=w242:u32)  [unwired: 1 in]
                    }
                    frame #1 {
                      w254 = T9 1 items=["FEATURE_FLAG_PRESENCE                 0x00000001", "FEATURE_FLAG_MANUAL                     0x00000002", "FEATURE_FLAG_AUTO                         0x00000004", "FEATURE_FLAG_ONEPUSH                   0x00000008", "FEATURE_FLAG_OFF                            0x00000010", "FEATURE_FLAG_DESC_SUPPORTED    0x00000020", "FEATURE_FLAG_READ_ONLY               0x00000040"] ("uFlags IN")
                      w255 = T10 8 items=["FEATURE_BRIGHTNESS", "FEATURE_EXPOSURE", "FEATURE_SHARPNESS", "FEATURE_WHITE_BAL", "FEATURE_HUE", "FEATURE_SATURATION", "FEATURE_GAMMA", "FEATURE_SHUTTER", "FEATURE_GAIN", "FEATURE_IRIS", "FEATURE_FOCUS", "FEATURE_TEMPERATURE", "FEATURE_TRIGGER", "FEATURE_ZOOM", "FEATURE_PAN", "FEATURE_TILT", "FEATURE_OPT_FILTER", "FEATURE_GPIO", "FEATURE_FRAME_RATE", "FEATURE_ROI", "FEATURE_FLIP", "FEATURE_PIXEL_ADDRESSING", "FEATURE_PIXEL_FORMAT", "FEATURE_EXTENDED_SHUTTER", "FEATURE_AUTO_ROI", "FEATURE_LOOKUP_TABLE", "FEATURE_MEMORY_CHANNEL", "FEATURE_WHITE_SHADING", "FEATURE_ROTATE", "FEATURE_IMAGER_CLK_DIVISOR", "FEATURE_TRIG_WITH_CNTRLD_LIGHT", "FEATURE_MAX_PIXEL_SIZE"] ("uFeatureId IN")
                      n84 = call <vilib>:"MEPU-CameraFeatures-SetFeature.vi"("hCamera IN"=w257, "uFeatureId IN"=w255, "uFlags IN"=w254, "pParms IN"=w249, "Error IN"=w256) -> ("hCamera OUT"=w253:u32, "Error OUT"=w248:errorcluster)  [unwired: 8 in, 1 out]
                      n85 = call "showError.vi"("message"="Ocurrio un error con el Gain", "Error IN"=w248) -> ("Error OUT"=w247:errorcluster)  [unwired: 3 in]
                      n86 = call "getCameraParameters.vi"("Error IN"=w247, "hCamera IN"=w253) -> ("Error OUT"=w251:errorcluster, "Camera Parameters"=w250:T6, "hCamera OUT"=w252:u32)  [unwired: 1 in]
                      n87 = call "StartStopCamera.vi"("Error IN"=w251, "Camara ON?"=w260, "hCamera IN"=w252) -> ("Error OUT"=w258:errorcluster, "hCamera OUT"=w259:u32)  [unwired: 1 in]
                    }
                  }
                  n88 = Unbundle By Name(w232) -> ("Stream?"=w234:bool, "Camera Parameters.Gain (dB)"=w231:dbl)
                  n89 = Build Array(w231) -> (w228:dbl[])
                  n90 = To Double Precision Float(number=w228) -> (double precision float=w227:dbl[])
                  n91 = Bundle By Name(cluster=w232, "Camera Parameters"=w230) -> (w233:T4)
                  n92 = call "camera2cluster.vi"("uSerialNumber IN"=w224, "Error IN"=w235, "hCamera IN"=w236) -> ("Camera Device OUT"=w226:T1)
                }
                frame "Saturation (%)" {
                  n93 = call "cluster2camera.vi"("Camera Device IN"=w262) -> ("Error OUT"=w274:errorcluster, "hCamera OUT"=w275:u32, "uSerialNumber OUT"=w261:u32)  [unwired: 2 in]
                  n94 = flat-sequence {
                    tunnel: w275 -> [w281]
                    tunnel: w274 -> [w280]
                    tunnel: [w279] -> w277
                    tunnel: [w278] -> w276
                    tunnel: w271 -> [w297]
                    tunnel: [w296] -> w273
                    tunnel: [w295] -> w272
                    tunnel: w277 -> [w294]
                    tunnel: w276 -> [w293]
                    tunnel: [w287] -> w267
                    tunnel: w264 -> [w286]
                    frame #0 {
                      n95 = call "StartStopCamera.vi"("Error IN"=w280, "Camara ON?"=FALSE, "hCamera IN"=w281) -> ("Error OUT"=w278:errorcluster, "hCamera OUT"=w279:u32)  [unwired: 1 in]
                    }
                    frame #1 {
                      w291 = T9 1 items=["FEATURE_FLAG_PRESENCE                 0x00000001", "FEATURE_FLAG_MANUAL                     0x00000002", "FEATURE_FLAG_AUTO                         0x00000004", "FEATURE_FLAG_ONEPUSH                   0x00000008", "FEATURE_FLAG_OFF                            0x00000010", "FEATURE_FLAG_DESC_SUPPORTED    0x00000020", "FEATURE_FLAG_READ_ONLY               0x00000040"] ("uFlags IN")
                      w292 = T10 5 items=["FEATURE_BRIGHTNESS", "FEATURE_EXPOSURE", "FEATURE_SHARPNESS", "FEATURE_WHITE_BAL", "FEATURE_HUE", "FEATURE_SATURATION", "FEATURE_GAMMA", "FEATURE_SHUTTER", "FEATURE_GAIN", "FEATURE_IRIS", "FEATURE_FOCUS", "FEATURE_TEMPERATURE", "FEATURE_TRIGGER", "FEATURE_ZOOM", "FEATURE_PAN", "FEATURE_TILT", "FEATURE_OPT_FILTER", "FEATURE_GPIO", "FEATURE_FRAME_RATE", "FEATURE_ROI", "FEATURE_FLIP", "FEATURE_PIXEL_ADDRESSING", "FEATURE_PIXEL_FORMAT", "FEATURE_EXTENDED_SHUTTER", "FEATURE_AUTO_ROI", "FEATURE_LOOKUP_TABLE", "FEATURE_MEMORY_CHANNEL", "FEATURE_WHITE_SHADING", "FEATURE_ROTATE", "FEATURE_IMAGER_CLK_DIVISOR", "FEATURE_TRIG_WITH_CNTRLD_LIGHT", "FEATURE_MAX_PIXEL_SIZE"] ("uFeatureId IN")
                      n96 = call <vilib>:"MEPU-CameraFeatures-SetFeature.vi"("hCamera IN"=w294, "uFeatureId IN"=w292, "uFlags IN"=w291, "pParms IN"=w286, "Error IN"=w293) -> ("hCamera OUT"=w290:u32, "Error OUT"=w285:errorcluster)  [unwired: 8 in, 1 out]
                      n97 = call "showError.vi"("message"="Ocurrio un error con el Saturation", "Error IN"=w285) -> ("Error OUT"=w284:errorcluster)  [unwired: 3 in]
                      n98 = call "getCameraParameters.vi"("Error IN"=w284, "hCamera IN"=w290) -> ("Error OUT"=w288:errorcluster, "Camera Parameters"=w287:T6, "hCamera OUT"=w289:u32)  [unwired: 1 in]
                      n99 = call "StartStopCamera.vi"("Error IN"=w288, "Camara ON?"=w297, "hCamera IN"=w289) -> ("Error OUT"=w295:errorcluster, "hCamera OUT"=w296:u32)  [unwired: 1 in]
                    }
                  }
                  n100 = Unbundle By Name(w269) -> ("Stream?"=w271:bool, "Camera Parameters.Saturation (%)"=w268:dbl)
                  n101 = Build Array(w268) -> (w265:dbl[])
                  n102 = To Double Precision Float(number=w265) -> (double precision float=w264:dbl[])
                  n103 = Bundle By Name(cluster=w269, "Camera Parameters"=w267) -> (w270:T4)
                  n104 = call "camera2cluster.vi"("uSerialNumber IN"=w261, "Error IN"=w272, "hCamera IN"=w273) -> ("Camera Device OUT"=w263:T1)
                }
                frame "Brightness (%)" {
                  n105 = call "cluster2camera.vi"("Camera Device IN"=w299) -> ("Error OUT"=w311:errorcluster, "hCamera OUT"=w312:u32, "uSerialNumber OUT"=w298:u32)  [unwired: 2 in]
                  n106 = flat-sequence {
                    tunnel: w312 -> [w318]
                    tunnel: w311 -> [w317]
                    tunnel: [w316] -> w314
                    tunnel: [w315] -> w313
                    tunnel: w310 -> [w334]
                    tunnel: [w333] -> w302
                    tunnel: [w332] -> w301
                    tunnel: w314 -> [w331]
                    tunnel: w313 -> [w330]
                    tunnel: [w324] -> w306
                    tunnel: w303 -> [w323]
                    frame #0 {
                      n107 = call "StartStopCamera.vi"("Error IN"=w317, "Camara ON?"=FALSE, "hCamera IN"=w318) -> ("Error OUT"=w315:errorcluster, "hCamera OUT"=w316:u32)  [unwired: 1 in]
                    }
                    frame #1 {
                      w328 = T9 1 items=["FEATURE_FLAG_PRESENCE                 0x00000001", "FEATURE_FLAG_MANUAL                     0x00000002", "FEATURE_FLAG_AUTO                         0x00000004", "FEATURE_FLAG_ONEPUSH                   0x00000008", "FEATURE_FLAG_OFF                            0x00000010", "FEATURE_FLAG_DESC_SUPPORTED    0x00000020", "FEATURE_FLAG_READ_ONLY               0x00000040"] ("uFlags IN")
                      w329 = T10 0 items=["FEATURE_BRIGHTNESS", "FEATURE_EXPOSURE", "FEATURE_SHARPNESS", "FEATURE_WHITE_BAL", "FEATURE_HUE", "FEATURE_SATURATION", "FEATURE_GAMMA", "FEATURE_SHUTTER", "FEATURE_GAIN", "FEATURE_IRIS", "FEATURE_FOCUS", "FEATURE_TEMPERATURE", "FEATURE_TRIGGER", "FEATURE_ZOOM", "FEATURE_PAN", "FEATURE_TILT", "FEATURE_OPT_FILTER", "FEATURE_GPIO", "FEATURE_FRAME_RATE", "FEATURE_ROI", "FEATURE_FLIP", "FEATURE_PIXEL_ADDRESSING", "FEATURE_PIXEL_FORMAT", "FEATURE_EXTENDED_SHUTTER", "FEATURE_AUTO_ROI", "FEATURE_LOOKUP_TABLE", "FEATURE_MEMORY_CHANNEL", "FEATURE_WHITE_SHADING", "FEATURE_ROTATE", "FEATURE_IMAGER_CLK_DIVISOR", "FEATURE_TRIG_WITH_CNTRLD_LIGHT", "FEATURE_MAX_PIXEL_SIZE"] ("uFeatureId IN")
                      n108 = call <vilib>:"MEPU-CameraFeatures-SetFeature.vi"("hCamera IN"=w331, "uFeatureId IN"=w329, "uFlags IN"=w328, "pParms IN"=w323, "Error IN"=w330) -> ("hCamera OUT"=w327:u32, "Error OUT"=w322:errorcluster)  [unwired: 8 in, 1 out]
                      n109 = call "showError.vi"("message"="Ocurrio un error con el Brightness", "Error IN"=w322) -> ("Error OUT"=w321:errorcluster)  [unwired: 3 in]
                      n110 = call "getCameraParameters.vi"("Error IN"=w321, "hCamera IN"=w327) -> ("Error OUT"=w325:errorcluster, "Camera Parameters"=w324:T6, "hCamera OUT"=w326:u32)  [unwired: 1 in]
                      n111 = call "StartStopCamera.vi"("Error IN"=w325, "Camara ON?"=w334, "hCamera IN"=w326) -> ("Error OUT"=w332:errorcluster, "hCamera OUT"=w333:u32)  [unwired: 1 in]
                    }
                  }
                  n112 = Unbundle By Name(w308) -> ("Stream?"=w310:bool, "Camera Parameters.Brightness (%)"=w307:dbl)
                  n113 = Build Array(w307) -> (w304:dbl[])
                  n114 = To Double Precision Float(number=w304) -> (double precision float=w303:dbl[])
                  n115 = Bundle By Name(cluster=w308, "Camera Parameters"=w306) -> (w309:T4)
                  n116 = call "camera2cluster.vi"("uSerialNumber IN"=w298, "Error IN"=w301, "hCamera IN"=w302) -> ("Camera Device OUT"=w300:T1)
                }
                frame "Pixel Format" {
                  n117 = call "cluster2camera.vi"("Camera Device IN"=w336) -> ("Error OUT"=w348:errorcluster, "hCamera OUT"=w349:u32, "uSerialNumber OUT"=w335:u32)  [unwired: 2 in]
                  n118 = flat-sequence {
                    tunnel: w349 -> [w355]
                    tunnel: w348 -> [w354]
                    tunnel: [w353] -> w351
                    tunnel: [w352] -> w350
                    tunnel: w345 -> [w371]
                    tunnel: [w370] -> w347
                    tunnel: [w369] -> w346
                    tunnel: w351 -> [w368]
                    tunnel: w350 -> [w367]
                    tunnel: [w361] -> w341
                    tunnel: w338 -> [w360]
                    frame #0 {
                      n119 = call "StartStopCamera.vi"("Error IN"=w354, "Camara ON?"=FALSE, "hCamera IN"=w355) -> ("Error OUT"=w352:errorcluster, "hCamera OUT"=w353:u32)  [unwired: 1 in]
                    }
                    frame #1 {
                      w365 = T9 1 items=["FEATURE_FLAG_PRESENCE                 0x00000001", "FEATURE_FLAG_MANUAL                     0x00000002", "FEATURE_FLAG_AUTO                         0x00000004", "FEATURE_FLAG_ONEPUSH                   0x00000008", "FEATURE_FLAG_OFF                            0x00000010", "FEATURE_FLAG_DESC_SUPPORTED    0x00000020", "FEATURE_FLAG_READ_ONLY               0x00000040"] ("uFlags IN")
                      w366 = T10 22 items=["FEATURE_BRIGHTNESS", "FEATURE_EXPOSURE", "FEATURE_SHARPNESS", "FEATURE_WHITE_BAL", "FEATURE_HUE", "FEATURE_SATURATION", "FEATURE_GAMMA", "FEATURE_SHUTTER", "FEATURE_GAIN", "FEATURE_IRIS", "FEATURE_FOCUS", "FEATURE_TEMPERATURE", "FEATURE_TRIGGER", "FEATURE_ZOOM", "FEATURE_PAN", "FEATURE_TILT", "FEATURE_OPT_FILTER", "FEATURE_GPIO", "FEATURE_FRAME_RATE", "FEATURE_ROI", "FEATURE_FLIP", "FEATURE_PIXEL_ADDRESSING", "FEATURE_PIXEL_FORMAT", "FEATURE_EXTENDED_SHUTTER", "FEATURE_AUTO_ROI", "FEATURE_LOOKUP_TABLE", "FEATURE_MEMORY_CHANNEL", "FEATURE_WHITE_SHADING", "FEATURE_ROTATE", "FEATURE_IMAGER_CLK_DIVISOR", "FEATURE_TRIG_WITH_CNTRLD_LIGHT", "FEATURE_MAX_PIXEL_SIZE"] ("uFeatureId IN")
                      n120 = call <vilib>:"MEPU-CameraFeatures-SetFeature.vi"("hCamera IN"=w368, "uFeatureId IN"=w366, "uFlags IN"=w365, "pParms IN"=w360, "Error IN"=w367) -> ("hCamera OUT"=w364:u32, "Error OUT"=w359:errorcluster)  [unwired: 8 in, 1 out]
                      n121 = call "showError.vi"("message"="Ocurrio un error con el Pixel Format", "Error IN"=w359) -> ("Error OUT"=w358:errorcluster)  [unwired: 3 in]
                      n122 = call "getCameraParameters.vi"("Error IN"=w358, "hCamera IN"=w364) -> ("Error OUT"=w362:errorcluster, "Camera Parameters"=w361:T6, "hCamera OUT"=w363:u32)  [unwired: 1 in]
                      n123 = call "StartStopCamera.vi"("Error IN"=w362, "Camara ON?"=w371, "hCamera IN"=w363) -> ("Error OUT"=w369:errorcluster, "hCamera OUT"=w370:u32)  [unwired: 1 in]
                    }
                  }
                  n124 = Unbundle By Name(w343) -> ("Stream?"=w345:bool, "Camera Parameters.Pixel Format"=w342:T3)
                  n125 = Build Array(w342) -> (w339:T3[])
                  n126 = To Double Precision Float(number=w339) -> (double precision float=w338:dbl[])
                  n127 = Bundle By Name(cluster=w343, "Camera Parameters"=w341) -> (w344:T4)
                  n128 = call "camera2cluster.vi"("uSerialNumber IN"=w335, "Error IN"=w346, "hCamera IN"=w347) -> ("Camera Device OUT"=w337:T1)
                }
                frame "Color Temperature (%)" {
                  n129 = call "cluster2camera.vi"("Camera Device IN"=w374) -> ("Error OUT"=w385:errorcluster, "hCamera OUT"=w386:u32, "uSerialNumber OUT"=w373:u32)  [unwired: 2 in]
                  n130 = Unbundle By Name(w380) -> ("Stream?"=w382:bool, "Camera Parameters.Color Temperature"=w379:dbl)
                  n131 = flat-sequence {
                    tunnel: w386 -> [w392]
                    tunnel: w385 -> [w391]
                    tunnel: [w390] -> w388
                    tunnel: [w389] -> w387
                    tunnel: w382 -> [w408]
                    tunnel: [w407] -> w384
                    tunnel: [w406] -> w383
                    tunnel: w388 -> [w405]
                    tunnel: w387 -> [w404]
                    tunnel: [w398] -> w378
                    tunnel: w375 -> [w397]
                    frame #0 {
                      n132 = call "StartStopCamera.vi"("Error IN"=w391, "Camara ON?"=FALSE, "hCamera IN"=w392) -> ("Error OUT"=w389:errorcluster, "hCamera OUT"=w390:u32)  [unwired: 1 in]
                    }
                    frame #1 {
                      w402 = T9 1 items=["FEATURE_FLAG_PRESENCE                 0x00000001", "FEATURE_FLAG_MANUAL                     0x00000002", "FEATURE_FLAG_AUTO                         0x00000004", "FEATURE_FLAG_ONEPUSH                   0x00000008", "FEATURE_FLAG_OFF                            0x00000010", "FEATURE_FLAG_DESC_SUPPORTED    0x00000020", "FEATURE_FLAG_READ_ONLY               0x00000040"] ("uFlags IN")
                      w403 = T10 11 items=["FEATURE_BRIGHTNESS", "FEATURE_EXPOSURE", "FEATURE_SHARPNESS", "FEATURE_WHITE_BAL", "FEATURE_HUE", "FEATURE_SATURATION", "FEATURE_GAMMA", "FEATURE_SHUTTER", "FEATURE_GAIN", "FEATURE_IRIS", "FEATURE_FOCUS", "FEATURE_TEMPERATURE", "FEATURE_TRIGGER", "FEATURE_ZOOM", "FEATURE_PAN", "FEATURE_TILT", "FEATURE_OPT_FILTER", "FEATURE_GPIO", "FEATURE_FRAME_RATE", "FEATURE_ROI", "FEATURE_FLIP", "FEATURE_PIXEL_ADDRESSING", "FEATURE_PIXEL_FORMAT", "FEATURE_EXTENDED_SHUTTER", "FEATURE_AUTO_ROI", "FEATURE_LOOKUP_TABLE", "FEATURE_MEMORY_CHANNEL", "FEATURE_WHITE_SHADING", "FEATURE_ROTATE", "FEATURE_IMAGER_CLK_DIVISOR", "FEATURE_TRIG_WITH_CNTRLD_LIGHT", "FEATURE_MAX_PIXEL_SIZE"] ("uFeatureId IN")
                      n133 = call <vilib>:"MEPU-CameraFeatures-SetFeature.vi"("hCamera IN"=w405, "uFeatureId IN"=w403, "uFlags IN"=w402, "pParms IN"=w397, "Error IN"=w404) -> ("hCamera OUT"=w401:u32, "Error OUT"=w396:errorcluster)  [unwired: 8 in, 1 out]
                      n134 = call "showError.vi"("message"="Ocurrio un error con el Coor Tenperature", "Error IN"=w396) -> ("Error OUT"=w395:errorcluster)  [unwired: 3 in]
                      n135 = call "getCameraParameters.vi"("Error IN"=w395, "hCamera IN"=w401) -> ("Error OUT"=w399:errorcluster, "Camera Parameters"=w398:T6, "hCamera OUT"=w400:u32)  [unwired: 1 in]
                      n136 = call "StartStopCamera.vi"("Error IN"=w399, "Camara ON?"=w408, "hCamera IN"=w400) -> ("Error OUT"=w406:errorcluster, "hCamera OUT"=w407:u32)  [unwired: 1 in]
                    }
                  }
                  n137 = Build Array(w379) -> (w376:dbl[])
                  n138 = To Double Precision Float(number=w376) -> (double precision float=w375:dbl[])
                  n139 = Bundle By Name(cluster=w380, "Camera Parameters"=w378) -> (w381:T4)
                  n140 = call "camera2cluster.vi"("uSerialNumber IN"=w373, "Error IN"=w383, "hCamera IN"=w384) -> ("Camera Device OUT"=w372:T1)
                }
                frame "Selector" {
                  n141 = Unbundle By Name(w421) -> ("Selector"=w414:u16, "Stream?"=w413:bool)
                  n142 = call "cluster2camera.vi"("Camera Device IN"=w411) -> ("Error OUT"=w419:errorcluster, "hCamera OUT"=w420:u32, "uSerialNumber OUT"=w409:u32)  [unwired: 2 in]
                  n143 = flat-sequence {
                    tunnel: w420 -> [w424]
                    tunnel: w419 -> [w423]
                    tunnel: w412 -> [w434]
                    tunnel: [w430] -> w416
                    tunnel: w413 -> [w429]
                    tunnel: [w427] -> w418
                    tunnel: [w426] -> w417
                    frame #0 {
                      n144 = call "StartStopCamera.vi"("Error IN"=w423, "Camara ON?"=FALSE, "hCamera IN"=w424) -> ()  [unwired: 1 in, 2 out]
                    }
                    frame #1 {
                      n145 = call <vilib>:"MEPU-Initialization-Initialize.vi"("uSerialNumber IN"=w434) -> ("phCamera OUT"=w433:u32, "Error OUT"=w432:errorcluster)  [unwired: 12 in, 1 out]
                      n146 = call "getCameraParameters.vi"("Error IN"=w432, "hCamera IN"=w433) -> ("Error OUT"=w431:errorcluster, "Camera Parameters"=w430:T6, "hCamera OUT"=w428:u32)  [unwired: 1 in]
                      n147 = call "StartStopCamera.vi"("Error IN"=w431, "Camara ON?"=w429, "hCamera IN"=w428) -> ("Error OUT"=w426:errorcluster, "hCamera OUT"=w427:u32)  [unwired: 1 in]
                    }
                  }
                  n148 = Index Array(array=w415, index=w414) -> (element=w412:u32)
                  n149 = Bundle By Name(cluster=w421, "Camera Parameters"=w416) -> (w422:T4)
                  n150 = call "camera2cluster.vi"("uSerialNumber IN"=w409, "Error IN"=w417, "hCamera IN"=w418) -> ("Camera Device OUT"=w410:T1)
                }
                frame "Stream" {
                  n151 = Unbundle By Name(w443) -> ("Stream?"=w438:bool)
                  n152 = call "cluster2camera.vi"("Camera Device IN"=w437) -> ("Error OUT"=w441:errorcluster, "hCamera OUT"=w442:u32, "uSerialNumber OUT"=w435:u32)  [unwired: 2 in]
                  n153 = call "StartStopCamera.vi"("Error IN"=w441, "Camara ON?"=w438, "hCamera IN"=w442) -> ("Error OUT"=w439:errorcluster, "hCamera OUT"=w440:u32)  [unwired: 1 in]
                  n154 = call "camera2cluster.vi"("uSerialNumber IN"=w435, "Error IN"=w439, "hCamera IN"=w440) -> ("Camera Device OUT"=w436:T1)
                }
                frame "Nothing", Default {
                }
              }
            }
          }
        }
      }
    }
  }
  "Camera Device OUT" <- w1
  n155 = Unbundle By Name(w12) -> ("Camera Parameters"=w11:T5, "Stream?"=w5:bool)
  "Stream? OUT" <- w5
  n156 = property class="Clust (strict)"(reference="Camera Parameters", "Value"=w11) -> ()  [unwired: 1 in, 2 out]
  n157 = property class="Bool (strict)"(reference="Stream?", "Value"=w5) -> ()  [unwired: 1 in, 2 out]
